vi "Get Alias.vi"(8 "error in (no error)":errorcluster, 11 "Multi Data in":refnum<class "Multi Data.lvclass">) -> (0 "error out":errorcluster, 2 "Alias":string, 3 "Multi Data out":refnum<class "Multi Data.lvclass">)   [LabVIEW 2020, in "Publisher.lvlib" / "Multi Data.lvclass"]
doc: "Return the Alias of the Data class.\n\nThis implementation returns the Alias from the private data if it isn't empty. If empty the parent method is called."
uses:
  Multi Data.lvclass
  Multi Data.lvclass/Multi Data.ctl
  Timed Data/Timed Data.lvclass
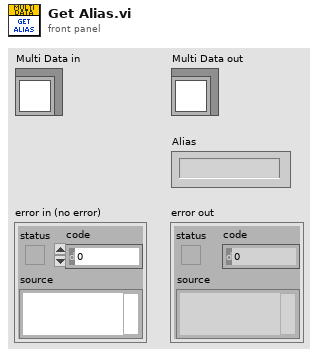
[diagram p1: front panel]
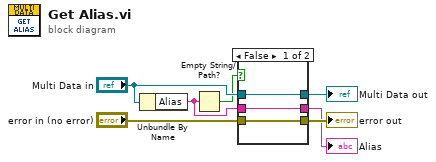
[diagram p0: block diagram]
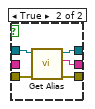
[diagram p2: hidden frame]
diagram:
  n1 = Unbundle By Name("Multi Data in") -> ("Alias"=w1:string)
  n2 = Empty String/Path?(string/path=w1) -> (empty?=w2:bool)
  n3 = case shown="False" w2 {
    tunnel: [w9 w15] -> w7
    tunnel: [w10 w14] -> w6
    tunnel: [w8 w13] -> w5
    tunnel: "error in (no error)" -> [w9 w12]
    tunnel: "Multi Data in" -> [w8 w11]
    tunnel: w1 -> [w10 _]
    frame False {
    }
    frame True {
      n4 = call-parent "Get Alias.vi"("error in (no error)"=w12, "Data in"=w11) -> ("error out"=w15:errorcluster, "Alias"=w14:string, "Data out"=w13:refnum<class "Multi Data.lvclass">)  [unwired: 7 in]
    }
  }
  "error out" <- w7
  "Multi Data out" <- w5
  "Alias" <- w6
